vi "SetParam.vi"(8 "error in (no error)":errorcluster caption="entrée d'erreur (pas d'erreur)", 10 "Binarizer":cluster{"threshold":dbl, "copy":bool}={"threshold"=0.0, "copy"=TRUE}, 11 "Binarizer en entrée":refnum<class "Binarizer.lvclass">) -> (0 "error out":errorcluster caption="sortie d'erreur", 3 "Binarizer en sortie":refnum<class "Binarizer.lvclass">)   [LabVIEW 2020, in "Binarizer.lvclass"]
doc: "Set Parameters"
uses:
  Binarizer.lvclass
  Binarizer.lvclass/Binarizer.ctl
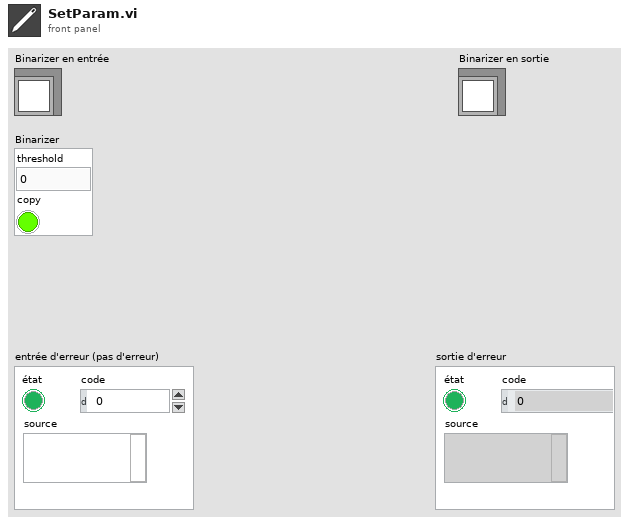
[diagram p1: front panel]
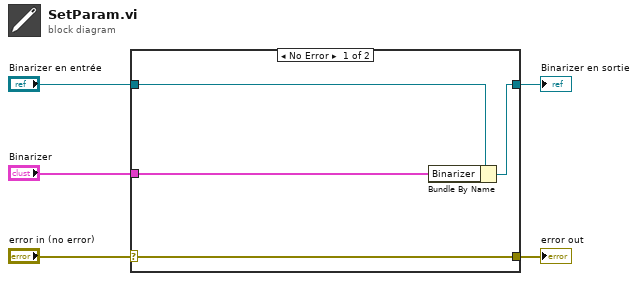
[diagram p0: block diagram]
diagram:
  n1 = case shown="No Error" "error in (no error)" {
    selector: "error in (no error)" -> [w9 w10]
    tunnel: [w9 w10] -> w4
    tunnel: [w7 w11] -> w2
    tunnel: "Binarizer en entrée" -> [w8 w11]
    tunnel: "Binarizer" -> [w6 _]
    frame No Error {
      n2 = Bundle By Name(cluster=w8, "Binarizer"=w6) -> (w7:refnum<class "Binarizer.lvclass">)
    }
    frame Error {
    }
  }
  "error out" <- w4
  "Binarizer en sortie" <- w2
